vi "Read_IR.vi"(0 "error in":errorcluster, 2 "Side":T2, 3 "node":string) -> (1 "error out":errorcluster, 4 "Range Data":T1)   [LabVIEW 2013]
doc: "Read the IR (either right or left)."
uses:
  ROS/Code/SubVIs/BaxterSide.ctl
panel:
  out "Reply":string
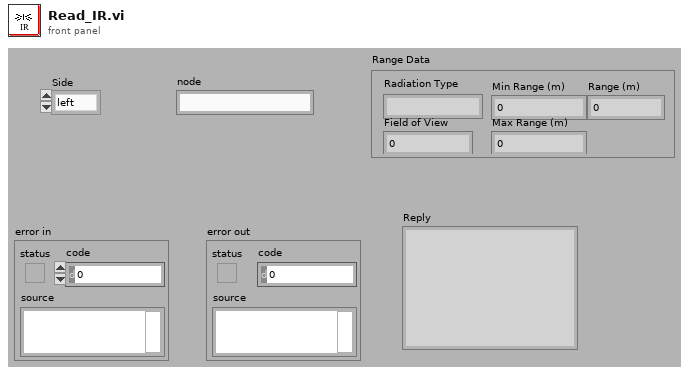
[diagram p1: front panel]
types:
  T1 = cluster{"Radiation Type":string, "Field of View":sgl, "Min Range (m)":sgl, "Max Range (m)":sgl, "Range (m)":sgl}
  T2 = typedef "BaxterSide.ctl" = enum16{"left", "right"}
  T3 = typedef "_ROSControl.ctl" = cluster{"topic port":u16, "Node":string, "topic":string, "type":string, "node port":u32, "error ":errorcluster, "Direction":T4, "APIs":string[]}
  T4 = typedef "_ROSDirection.ctl" = enum16{"Node", "Publisher", "Subscriber", "Service Client"}
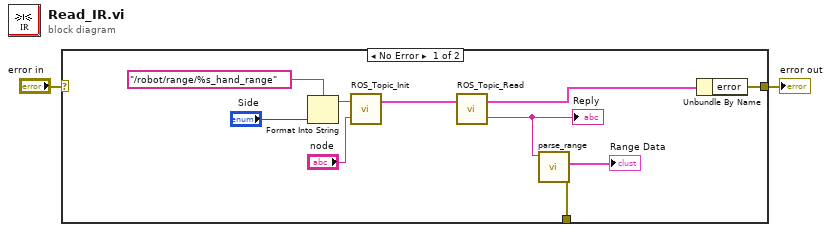
[diagram p0: block diagram]
diagram:
  n1 = case shown="No Error" "error in" {
    selector: "error in" -> [_ w13]
    tunnel: [w12 w13] -> w2
    tunnel: [w4 _] -> _
    frame No Error {
      n2 = Format Into String(format string="/robot/range/%s_hand_range" ("topic"), "Side") -> (resulting string=w7:string)  [unwired: 2 in, 1 out]
      n3 = call "ROS_Topic_Init.vi"("node"="node", "topic"=w7) -> ("ROS out"=w10:T3)  [unwired: 1 in]
      n4 = call "ROS_Topic_Read.vi"("ROS in"=w10) -> ("Reply"=w5:string, "ROS out"=w9:T3)  [unwired: 1 in]
      "Reply" <- w5
      n5 = call "parse_range.vi"("msg in"=w5) -> ("error out"=w4:errorcluster, "Range Data"=→"Range Data":T1)  [unwired: 3 in, 2 out]
      n6 = Unbundle By Name(w9) -> ("error"=w12:errorcluster)
    }
    frame Error {
    }
  }
  "error out" <- w2
